vi "Filter Messages by Direction.vi"(8 "error in":errorcluster, 10 "filtered direction":T1=enum."Tx", 11 "all messages and subaddresses":T2[](array[typedef]) {"Timestamp Channel Handle" format="%.0x"; "Message Section Handle" format="%.0x"; "Parameter Channel Handles" format="%.0x"}) -> (0 "error out":errorcluster, 2 "channel handles":T3[](array[typedef]) format="%.0x", 3 "filtered messages and subaddresses":T2[](array[typedef]) {"Timestamp Channel Handle" format="%.0x"; "Message Section Handle" format="%.0x"; "Parameter Channel Handles" format="%.0x"})   [LabVIEW 2020, in "AIM MIL-STD-1553 Engine.lvlib" / "Implementation.lvlib" / "Execution Unit.lvclass"]
uses:
  Execution Unit.lvclass
  Shared/Direction.ctl
  <vilib>/NI VeriStand/Custom Device API/Custom Device Item Ref.ctl
  <vilib>/NI VeriStand/Custom Device API/Custom Device API.lvlib
  Shared/Parameter Definition.ctl
  Custom Device/Compiled Message.ctl
  Custom Device/Custom Device.lvlib
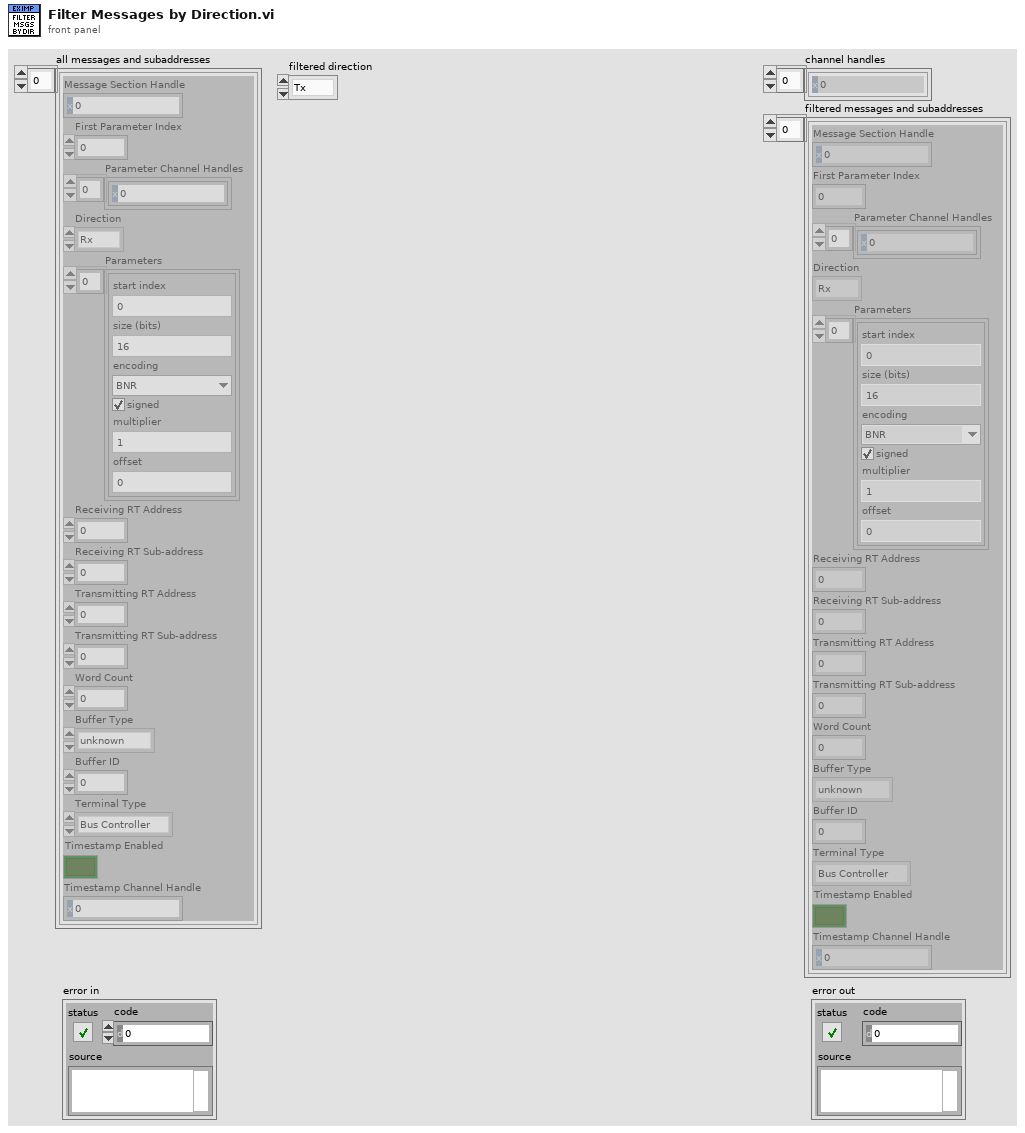
[diagram p1: front panel]
types:
  T1 = typedef "Direction.ctl" = enum16{"Rx", "Tx"}
  T2 = typedef "AIM MIL-STD-1553 Engine.lvlib/Custom Device.lvlib/Compiled Message.ctl" = cluster{"Message Section Handle":T3, "First Parameter Index":i32, "Parameter Channel Handles":T3[], "Direction":T1, "Parameters":T4[], "Receiving RT Address":u8, "Receiving RT Sub-address":u8, "Transmitting RT Address":u8, "Transmitting RT Sub-address":u8, "Word Count":u8, "Buffer Type":enum16{"unknown", "BC Message Buffer", "RT Message Buffer"}, "Buffer ID":u16, "Terminal Type":enum16{"Bus Controller", "Remote Terminal"}, "Timestamp Enabled":bool, "Timestamp Channel Handle":T3}
  T3 = typedef "Custom Device API.lvlib/Custom Device Item Ref.ctl" = u64
  T4 = typedef "Parameter Definition.ctl" = cluster{"start index":i32, "size (bits)":i32, "encoding":enum16{"BNR", "BCD", "Discrete"}, "signed":bool, "multiplier":dbl, "offset":dbl}
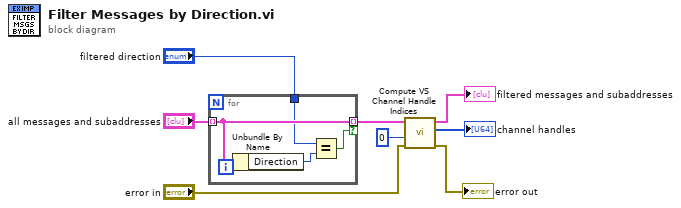
[diagram p0: block diagram]
diagram:
  n1 = for {
    tunnel: "all messages and subaddresses" -> [w12] mode=indexing
    tunnel: [w12] -> w7 mode=indexing if=w10
    tunnel: "filtered direction" -> [w9]
    n2 = Unbundle By Name(w12) -> ("Direction"=w11:T1)
    n3 = Equal?(x=w9, y=w11) -> (x = y?=w10:bool)
  }
  n4 = call "Compute VS Channel Handle Indices.vi"("error in (no error)"="error in", "next index"=0, "messages and subaddresses"=w7) -> ("error out"=→"error out":errorcluster, "channel handles"=→"channel handles":T3[], "messages and subaddresses out"=→"filtered messages and subaddresses":T2[])  [unwired: 5 in, 1 out]
